vi "ActiveXMediaPlayer.vi"() -> ()   [LabVIEW 2019]
panel:
  out "time string":string
  out "String":string
  in  "Seek Back Button":bool
  in  "Open Button":bool
  in  "Seek Forward Button":bool
  in  "MediaStopButton":bool
  in  "Pause Button":bool
  in  "Play Button":bool
  in  "WMP":refnum<k7>(container)
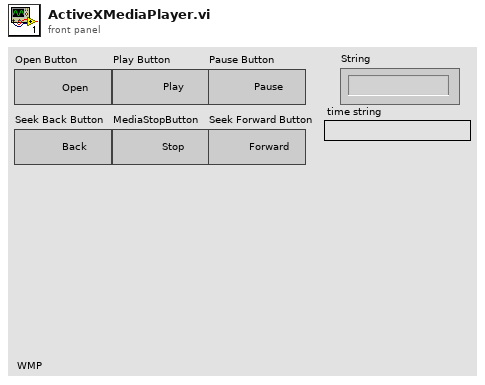
[diagram p1: front panel]
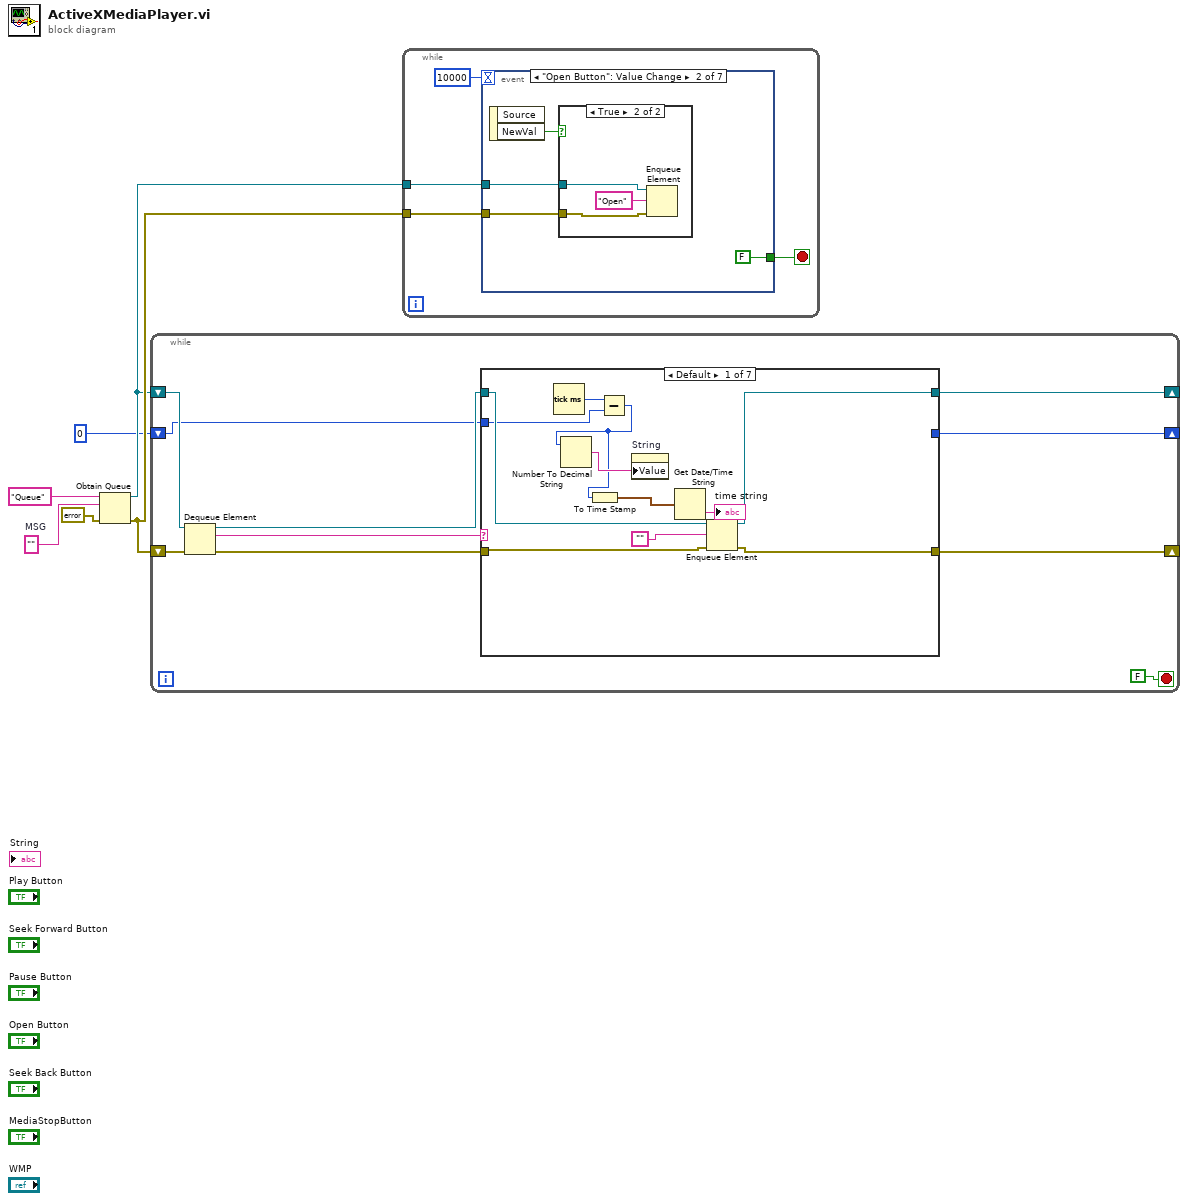
[diagram p0: block diagram]
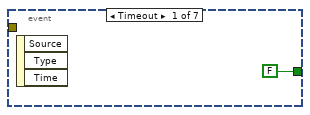
[diagram p2: hidden frame]
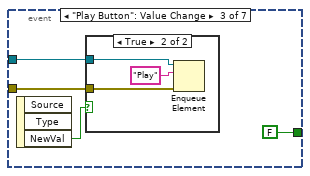
[diagram p4: hidden frame]
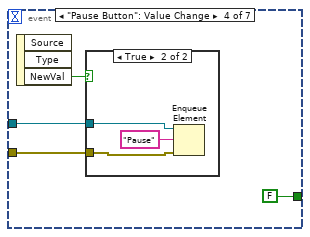
[diagram p6: hidden frame]
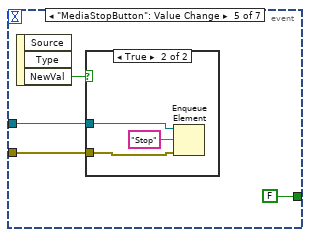
[diagram p8: hidden frame]
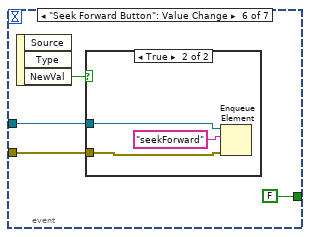
[diagram p10: hidden frame]
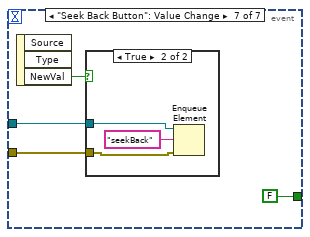
[diagram p12: hidden frame]
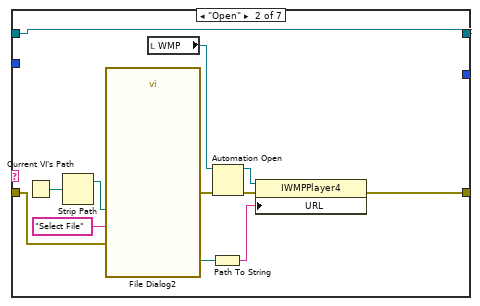
[diagram p14: hidden frame]
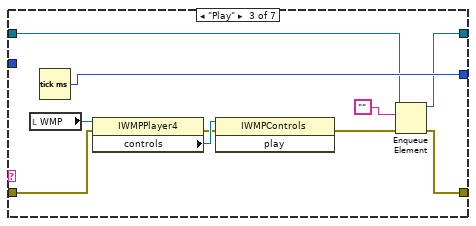
[diagram p15: hidden frame]
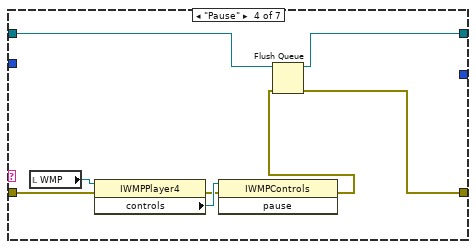
[diagram p16: hidden frame]
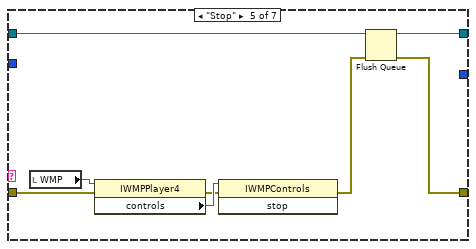
[diagram p17: hidden frame]
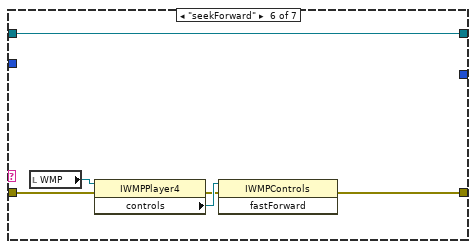
[diagram p18: hidden frame]
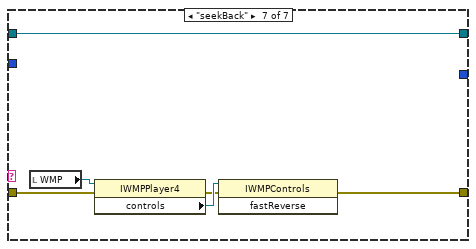
[diagram p19: hidden frame]
diagram:
  w2 = ""  # MSG
  n1 = Obtain Queue(name (unnamed)="Queue", element data type=w2, error in (no error)=errorcluster {"status"=FALSE, "code"=0, "source"=""}) -> (queue out=w3:refnum<queue>, error out=w5:errorcluster)  [unwired: 2 in, 1 out]
  n2 = while {
    shift-right: [w16] -> _
    shift-left: w5 -> [w11]
    shift-right: [w10] -> _
    shift-left: w3 -> [w12]
    shift-right: [w8] -> _
    shift-left: u32 0 ("millisecond timer value") -> [w7]
    stop <- FALSE stop-if-true
    n3 = Dequeue Element(queue=w12, error in (no error)=w11) -> (queue out=w14:refnum<queue>, element=w13:string, error out=w15:errorcluster)  [unwired: 1 in, 1 out]
    n4 = case shown="Default" w13 {
      tunnel: w15 -> [w27 w36 w48 w56 w64 w70 w76]
      tunnel: [w26 w31 w42 w50 w58 w67 w73] -> w16
      tunnel: w14 -> [w24 w28 w44 w53 w61 w66 w72]
      tunnel: [w23 w28 w41 w52 w60 w66 w72] -> w10
      tunnel: [_ _ w45 _ _ _ _] -> w8
      tunnel: w7 -> [w21 _ _ _ _ _ _]
      frame Default {
        n5 = Tick Count (ms)() -> (millisecond timer value=w22:u32)
        n6 = Subtract(x=w22, y=w21) -> (x-y=w19:u32)
        n7 = Number To Decimal String(number=w19) -> (decimal integer string=w20:string)  [unwired: 1 in]
        n8 = To Time Stamp(1:w19) -> (0:w18:timestamp)
        n9 = property on="String" class="Str"("Value"=w20) -> ()  [unwired: 2 in, 2 out]
        n10 = Get Date/Time String(seconds (now)=w18) -> (time string=→"time string":string)  [unwired: 2 in, 1 out]
        n11 = Enqueue Element(queue=w24, element="", error in (no error)=w27) -> (queue out=w23:refnum<queue>, error out=w26:errorcluster)  [unwired: 1 in, 1 out]
      }
      frame "Open" {
        n12 = Current VI's Path() -> (path=w39:path)
        n13 = Strip Path(path=w39) -> (stripped path=w38:path)  [unwired: 1 out]
        n14 = call "File Dialog2"("start path"=w38, "prompt"="Select File", "error in"=w36) -> ("selected path"=w33:path, "error out"=w32:errorcluster)  [unwired: 9 in, 2 out]
        n15 = local read "WMP"() -> (w30:refnum<k7>)
        n16 = Path To String(path=w33) -> (string=w34:string)
        n17 = Automation Open(error in (no error)=w32, Automation Refnum=w30) -> (Automation Refnum=w29:refnum<k7>, error out=w35:errorcluster)  [unwired: 2 in]
        n18 = property class="IWMPPlayer4"(reference=w29, error in=w35, "URL"=w34) -> (error out=w31:errorcluster)  [unwired: 1 out]
      }
      frame "Play" {
        n19 = local read "WMP"() -> (w49:refnum<k7>)
        n20 = Tick Count (ms)() -> (millisecond timer value=w45:u32)
        n21 = property class="IWMPPlayer4"(reference=w49, error in=w48) -> (error out=w46:errorcluster, "controls"=w47:refnum<k7>)  [unwired: 1 out]
        n22 = invoke class="IWMPControls" method="play"(reference=w47, error in=w46) -> (error out=w43:errorcluster)  [unwired: 1 in, 2 out]
        n23 = Enqueue Element(queue=w44, element="", error in (no error)=w43) -> (queue out=w41:refnum<queue>, error out=w42:errorcluster)  [unwired: 1 in, 1 out]
      }
      frame "Pause" {
        n24 = local read "WMP"() -> (w57:refnum<k7>)
        n25 = property class="IWMPPlayer4"(reference=w57, error in=w56) -> (error out=w54:errorcluster, "controls"=w55:refnum<k7>)  [unwired: 1 out]
        n26 = invoke class="IWMPControls" method="pause"(reference=w55, error in=w54) -> (error out=w51:errorcluster)  [unwired: 1 in, 2 out]
        n27 = Flush Queue(queue=w53, error in (no error)=w51) -> (queue out=w52:refnum<queue>, error out=w50:errorcluster)  [unwired: 1 out]
      }
      frame "Stop" {
        n28 = local read "WMP"() -> (w65:refnum<k7>)
        n29 = property class="IWMPPlayer4"(reference=w65, error in=w64) -> (error out=w62:errorcluster, "controls"=w63:refnum<k7>)  [unwired: 1 out]
        n30 = invoke class="IWMPControls" method="stop"(reference=w63, error in=w62) -> (error out=w59:errorcluster)  [unwired: 1 in, 2 out]
        n31 = Flush Queue(queue=w61, error in (no error)=w59) -> (queue out=w60:refnum<queue>, error out=w58:errorcluster)  [unwired: 1 out]
      }
      frame "seekForward" {
        n32 = local read "WMP"() -> (w71:refnum<k7>)
        n33 = property class="IWMPPlayer4"(reference=w71, error in=w70) -> (error out=w68:errorcluster, "controls"=w69:refnum<k7>)  [unwired: 1 out]
        n34 = invoke class="IWMPControls" method="fastForward"(reference=w69, error in=w68) -> (error out=w67:errorcluster)  [unwired: 1 in, 2 out]
      }
      frame "seekBack" {
        n35 = local read "WMP"() -> (w77:refnum<k7>)
        n36 = property class="IWMPPlayer4"(reference=w77, error in=w76) -> (error out=w74:errorcluster, "controls"=w75:refnum<k7>)  [unwired: 1 out]
        n37 = invoke class="IWMPControls" method="fastReverse"(reference=w75, error in=w74) -> (error out=w73:errorcluster)  [unwired: 1 in, 2 out]
      }
    }
  }
  n38 = while {
    tunnel: w5 -> [w81]
    tunnel: w3 -> [w80]
    stop <- w78 stop-if-true
    n39 = event shown="[1] \"Open Button\": Value Change" {
      selector: _ -> [_ _ _ _ _ _ _]
      dyn-events: _ -> [_ _ _ _ _ _ _]
      timeout: 10000 -> [_ _ _ _ _ _ _]
      tunnel: [FALSE FALSE FALSE FALSE FALSE FALSE FALSE] -> w78
      tunnel: w80 -> [_ w85 w92 w99 w106 w113 w120]
      tunnel: w81 -> [_ w84 w91 w98 w105 w112 w119]
      event Timeout {
        n40 = event-data() -> ()  [unwired: 1 in, 3 out]
      }
      event "Open Button": Value Change {
        n41 = event-data() -> ("NewVal"=w86:bool)  [unwired: 1 in, 1 out]
        n42 = case shown="True" w86 {
          tunnel: w85 -> [_ w89]
          tunnel: w84 -> [_ w88]
          frame False {
          }
          frame True {
            n43 = Enqueue Element(queue=w89, element="Open", error in (no error)=w88) -> ()  [unwired: 1 in, 3 out]
          }
        }
      }
      event "Play Button": Value Change {
        n44 = event-data() -> ("NewVal"=w90:bool)  [unwired: 1 in, 2 out]
        n45 = case shown="True" w90 {
          tunnel: w92 -> [_ w95]
          tunnel: w91 -> [_ w94]
          frame False {
          }
          frame True {
            n46 = Enqueue Element(queue=w95, element="Play", error in (no error)=w94) -> ()  [unwired: 1 in, 3 out]
          }
        }
      }
      event "Pause Button": Value Change {
        n47 = event-data() -> ("NewVal"=w97:bool)  [unwired: 1 in, 2 out]
        n48 = case shown="True" w97 {
          tunnel: w99 -> [_ w102]
          tunnel: w98 -> [_ w101]
          frame False {
          }
          frame True {
            n49 = Enqueue Element(queue=w102, element="Pause", error in (no error)=w101) -> ()  [unwired: 1 in, 3 out]
          }
        }
      }
      event "MediaStopButton": Value Change {
        n50 = event-data() -> ("NewVal"=w104:bool)  [unwired: 1 in, 2 out]
        n51 = case shown="True" w104 {
          tunnel: w106 -> [_ w109]
          tunnel: w105 -> [_ w108]
          frame False {
          }
          frame True {
            n52 = Enqueue Element(queue=w109, element="Stop", error in (no error)=w108) -> ()  [unwired: 1 in, 3 out]
          }
        }
      }
      event "Seek Forward Button": Value Change {
        n53 = event-data() -> ("NewVal"=w111:bool)  [unwired: 1 in, 2 out]
        n54 = case shown="True" w111 {
          tunnel: w113 -> [_ w116]
          tunnel: w112 -> [_ w115]
          frame False {
          }
          frame True {
            n55 = Enqueue Element(queue=w116, element="seekForward", error in (no error)=w115) -> ()  [unwired: 1 in, 3 out]
          }
        }
      }
      event "Seek Back Button": Value Change {
        n56 = event-data() -> ("NewVal"=w118:bool)  [unwired: 1 in, 2 out]
        n57 = case shown="True" w118 {
          tunnel: w120 -> [_ w123]
          tunnel: w119 -> [_ w122]
          frame False {
          }
          frame True {
            n58 = Enqueue Element(queue=w123, element="seekBack", error in (no error)=w122) -> ()  [unwired: 1 in, 3 out]
          }
        }
      }
    }
  }
